vi "Cycle End.vi"(8 "error in (no error)":errorcluster, 11 "Framework in":refnum<class "Framework.lvclass">) -> (0 "error out":errorcluster, 3 "Framework out":refnum<class "Framework.lvclass">)   [LabVIEW 2020, in "DSF Core.lvlib" / "Framework.lvclass"]
uses:
  Framework.lvclass
  Performance/Performance.lvclass
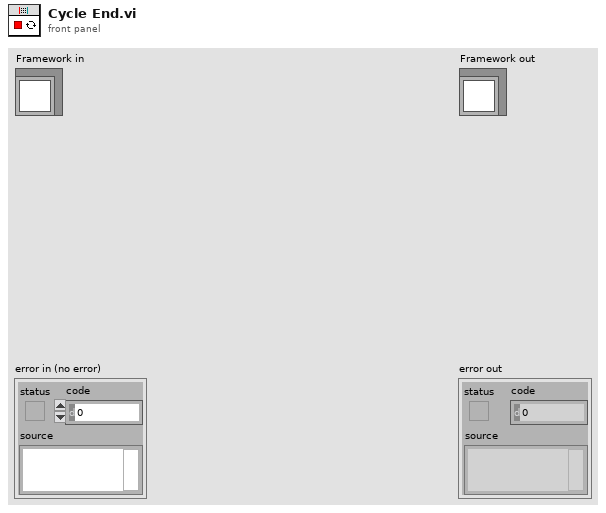
[diagram p1: front panel]
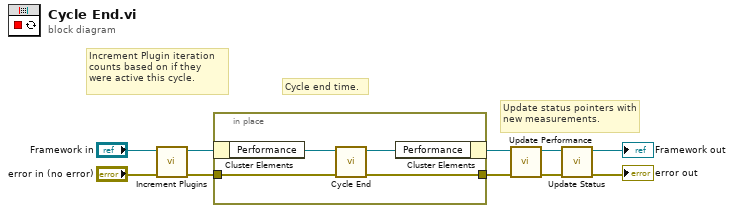
[diagram p0: block diagram]
diagram:
  # "Update status pointers with new measurements."
  # "Cycle end time."
  # "Increment Plugin iteration counts based on if they were active this cycle."
  n1 = call "Increment Plugins.vi"("error in (no error)"="error in (no error)", "Framework in"="Framework in") -> ("error out"=w1:errorcluster, "Framework out"=w2:refnum<class "Framework.lvclass">)  [unwired: 8 in]
  n2 = in-place {
    in-place-border: w1 -> [w12]
    in-place-border: [w11] -> w7
    n3 = in-place-cluster #1(w2) -> ("Performance"=w14:refnum<class "Performance.lvclass">)
    n4 = call "Cycle End.vi"("error in (no error)"=w12, "Performance in"=w14) -> ("error out"=w11:errorcluster, "Performance out"=w13:refnum<class "Performance.lvclass">)  [unwired: 8 in]
    n5 = in-place-cluster #1("Performance"=w13) -> (w8:refnum<class "Framework.lvclass">)
  }
  n6 = call "Update Performance.vi"("error in (no error)"=w7, "Framework in"=w8) -> ("error out"=w9:errorcluster, "Framework out"=w10:refnum<class "Framework.lvclass">)  [unwired: 8 in]
  n7 = call "Update Status.vi"("error in (no error)"=w9, "Framework in"=w10) -> ("error out"=→"error out":errorcluster, "Framework out"=→"Framework out":refnum<class "Framework.lvclass">)  [unwired: 8 in]
